vi "Apply Mask to Routing Channel.vi"(8 "error in (no error)":errorcluster, 10 "Mask":enum16{"Disable", "Enable"}(ring), 11 "Channel Ref in":T1 format="%.0x") -> (0 "error out":errorcluster, 3 "Channel Ref out":T1 format="%.0x")   [LabVIEW 2017, in "Routing and Faulting Scripting.lvlib"]
uses:
  Routing and Faulting Scripting.lvlib
  <vilib>/NI Veristand/Custom Device API/Custom Device Item Ref.ctl
  NationalInstruments.VeriStand.SystemDefinitionAPI
  NationalInstruments.VeriStand.SystemStorage
  <vilib>/NI Veristand/Custom Device API/Custom Device API.lvlib
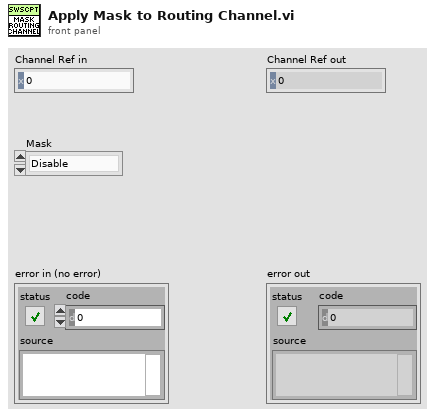
[diagram p1: front panel]
types:
  T1 = typedef "Custom Device API.lvlib/Custom Device Item Ref.ctl" = u64
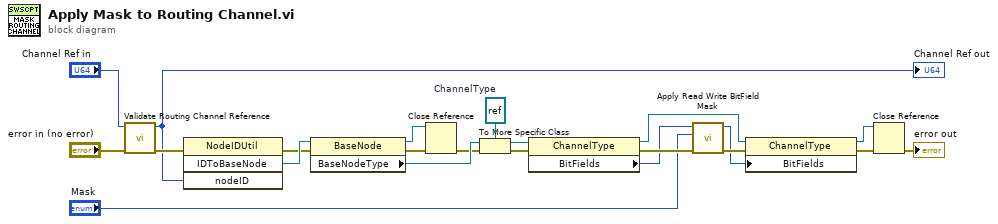
[diagram p0: block diagram]
diagram:
  w18 = refnum<k24> refnum  # ChannelType
  n1 = call "Validate Routing Channel Reference.vi"("error in (no error)"="error in (no error)", "Channel Ref in"="Channel Ref in") -> ("error out"=w21:errorcluster, "Channel Ref out"=w6:T1)  [unwired: 8 in]
  "Channel Ref out" <- w6
  n2 = invoke class="NodeIDUtil" method="IDToBaseNode"(error in=w21, "nodeID"=w6) -> (error out=w16:errorcluster, "IDToBaseNode"=w17:refnum<k24>)  [unwired: 2 in, 2 out]
  n3 = property class="BaseNode"(reference=w17, error in=w16) -> (reference out=w4:refnum<k24>, error out=w20:errorcluster, "BaseNodeType"=w19:refnum<k24>)
  n4 = Close Reference(reference=w4, error in (no error)=w20) -> (error out=w5:errorcluster)
  n5 = To More Specific Class(target class=w18, reference=w19, error in=w5) -> (specific class reference=w11:refnum<k24>, error out=w15:errorcluster)
  n6 = property class="ChannelType"(reference=w11, error in=w15) -> (reference out=w14:refnum<k24>, error out=w13:errorcluster, "BitFields"=w10:u32)
  n7 = call "Apply Read Write BitField Mask.vi"("error in (no error)"=w13, "Mask"="Mask", "BitFields in"=w10) -> ("error out"=w12:errorcluster, "BitFields out"=w9:u32)  [unwired: 7 in]
  n8 = property class="ChannelType"(reference=w14, error in=w12, "BitFields"=w9) -> (reference out=w2:refnum<k24>, error out=w7:errorcluster)
  n9 = Close Reference(reference=w2, error in (no error)=w7) -> (error out=→"error out":errorcluster)
